vi "set outputs.vi"(8 "error in":errorcluster, 9 "Timeout (ms)":i32=-1, 10 "output data":T1[](array[typedef]), 11 "profibus reference":T2) -> (0 "error out":errorcluster, 3 "profibus reference out":T2)   [LabVIEW 2013, in "dynamic profibus.lvlib"]
uses:
  dynamic profibus.lvlib
  fpga reference.ctl
  dataset.ctl
  <vilib>/rvi/interface/common/niFpgaWaitOnOcc.vi
  <vilib>/Utility/error.llb/Error Cluster From Error Code.vi
  <vilib>/rvi/errors/niLvFpgaAdjustHostInterfaceError.vi
  <vilib>/rvi/interface/nirviMethod/nirviMethod.xnode
  <vilib>/FPGAPlugInAG/Dynamic/niLvFpga_WriteFifo_Dynamic.vi
  <vilib>/rvi/errors/niLvFpgaMergeErrorWithErrorCode.vi
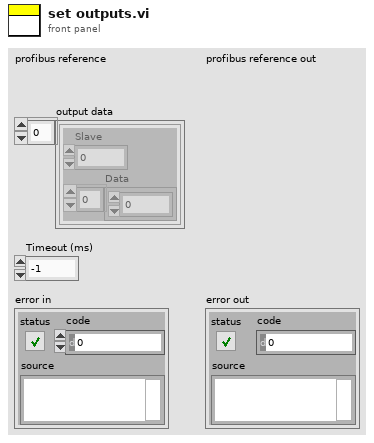
[diagram p1: front panel]
types:
  T1 = typedef "dynamic profibus.lvlib/dataset.ctl" = cluster{"Slave":u8, "Data":u8[]}
  T2 = typedef "dynamic profibus.lvlib/fpga reference.ctl" = refnum<k20>
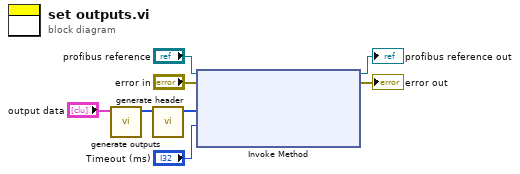
[diagram p0: block diagram]
diagram:
  n1 = call "generate outputs.vi"("output data"="output data") -> ("data array w/o header"=w3:u32[])  [unwired: 10 in]
  n2 = call "generate header.vi"("data in"=w3) -> ("data + header"=w2:u32[])  [unwired: 10 in]
  n3 = xnode "Invoke Method"("FPGA VI Reference In"="profibus reference", "error in"="error in", "Data"=w2, "Timeout (ms)"="Timeout (ms)") -> ("FPGA VI Reference Out"=→"profibus reference out":T2, "error out"=→"error out":errorcluster)  [unwired: 1 out]
